vi "acquire single wave by LAN.vi"() -> ()   [LabVIEW 2013]
panel:
  out "Waveform Graph":i32[](graph)
  in  "IP address":string="192.168.1.72"
  out "VOLTS/DIV":string
  in  "stop":bool
  out "SEC/DIV":string
  out "CH1":string
  out "probe":string
  out "scale":string
  # "1.Fill in the IP Address of your device"
  # "2.Please use the stop button to stop the vi"
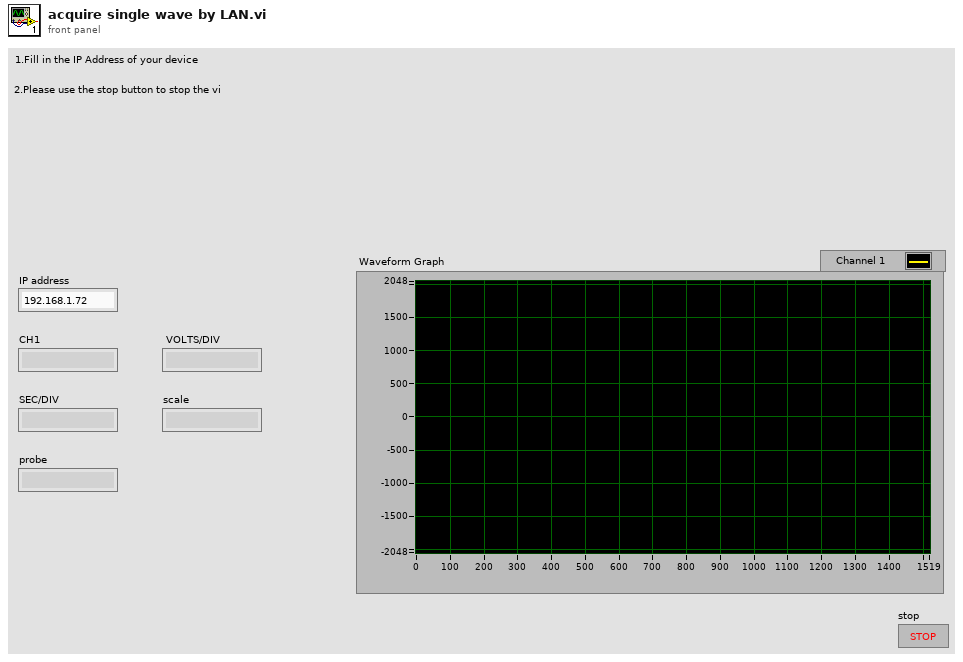
[diagram p1: front panel]
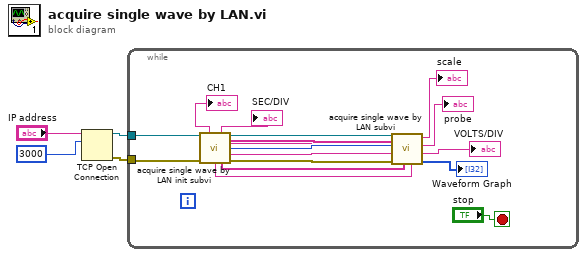
[diagram p0: block diagram]
diagram:
  n1 = TCP Open Connection(address="IP address", remote port or service name=u16 3000) -> (connection ID=w2:refnum<k5>, error out=w1:errorcluster)  [unwired: 3 in]
  n2 = while {
    tunnel: w2 -> [w13]
    tunnel: w1 -> [w12]
    stop <- "stop" stop-if-true
    n3 = call "acquire single wave by LAN init subvi.vi"("TCP Network Connection in"=w13, "error in (no error)"=w12) -> ("CH1"=→"CH1":string, "Array 3"=w18:string[], "SEC/DIV"=→"SEC/DIV":string, "TCP Network Connection out"=w20:refnum<k5>, "Array 2"=w17:string[], "Numeric"=w15:i32, "data out"=w11:string, "ID Query"=w14:string, "Array"=w16:string[], "error out"=w19:errorcluster)  [unwired: 4 in]
    n4 = call "acquire single wave by LAN subvi.vi"("ID Query"=w14, "Array 4"=w18, "Array in"=w16, "Array 3"=w17, "error in (no error)"=w19, "data in"=w11, "Numeric"=w15, "TCP Network Connection in"=w20) -> ("Array out"=→"Waveform Graph":i32[], "VOLTS/DIV"=→"VOLTS/DIV":string, "probe"=→"probe":string, "scale"=→"scale":string)
  }
